vi "Script Dyn-Conf.vi"(6 "error in (no error)":errorcluster, 7 "TDX":bool[](array[boolean]), 8 "DelayuS":i32=7, 9 "VISA resource name IN":refnum<visa-resource-name>) -> (0 "error out":errorcluster, 1 "Tamaño Script":i32, 2 "Orden Transd":u64, 3 "VISA resource name OUT":refnum<visa-resource-name>)   [LabVIEW 2014, in "CAP-USB.lvlib"]
doc: "Este VI arma un array de N elementos en donde cada elemento es una linea de configuracion que luego envia al CAP-USB pasa su configuracion."
uses:
  CAP-USB.lvlib
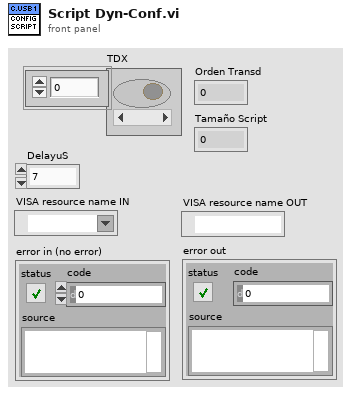
[diagram p1: front panel]
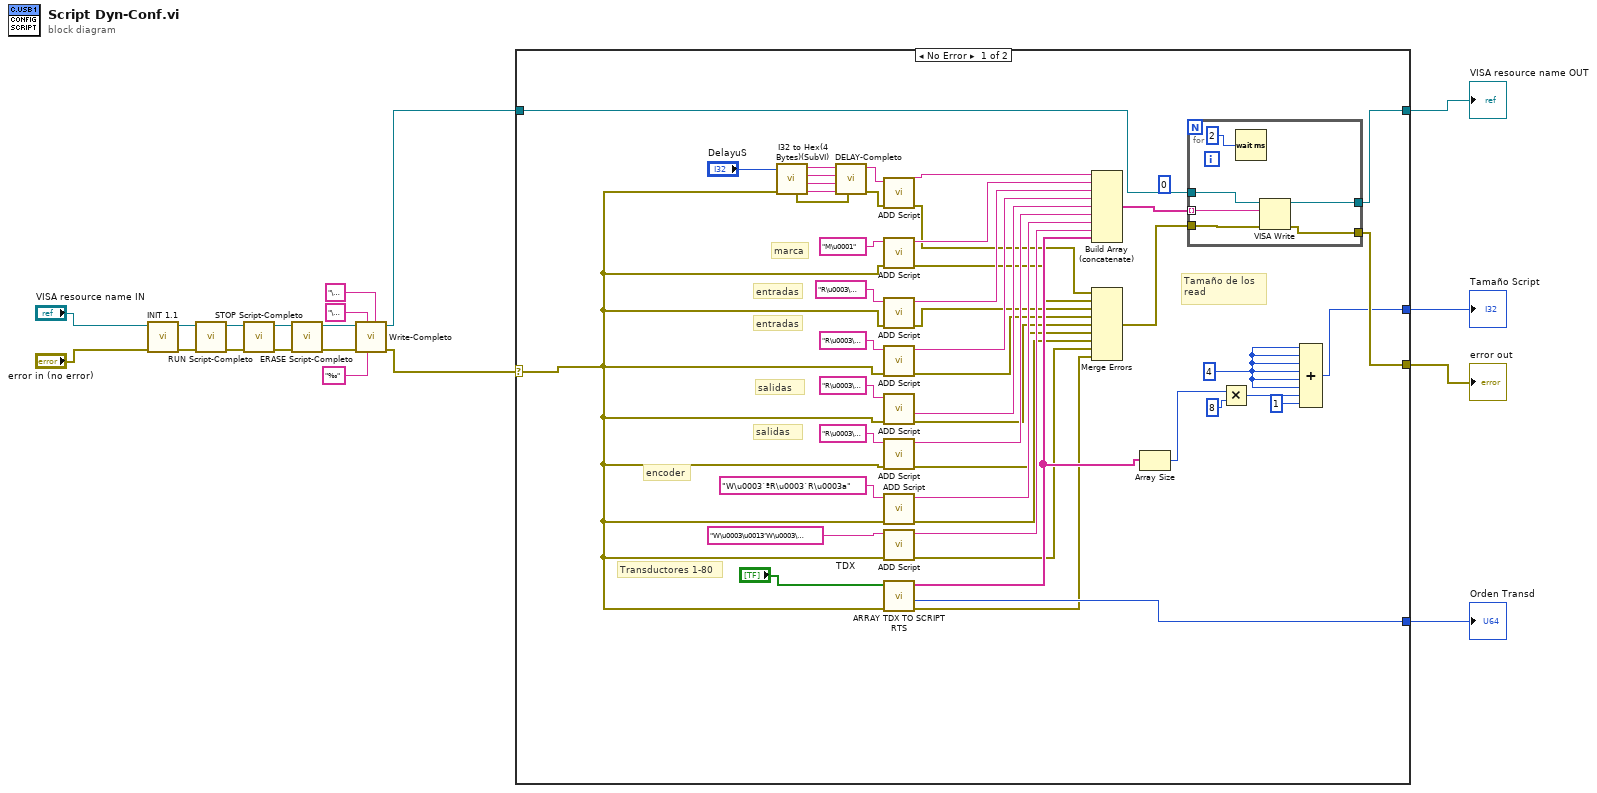
[diagram p0: block diagram]
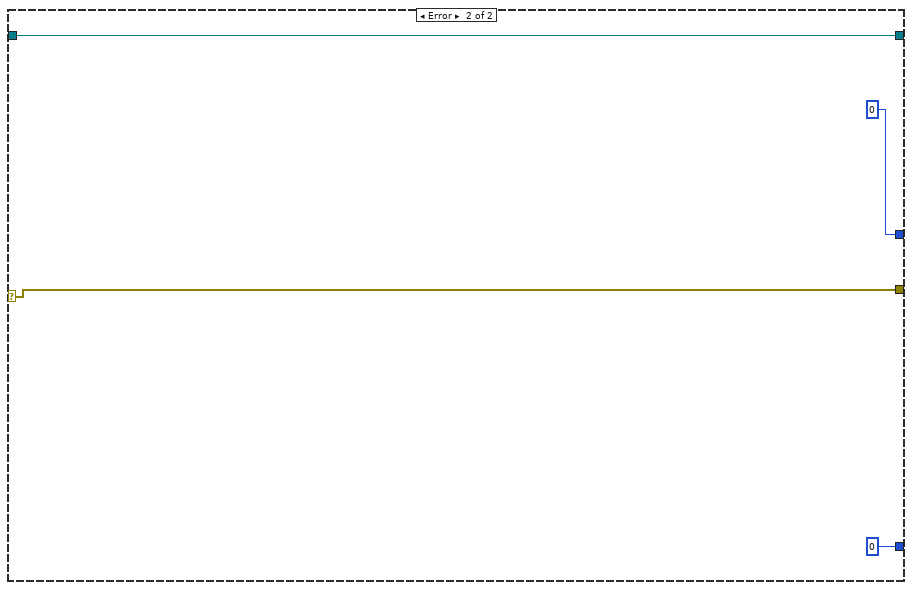
[diagram p2: hidden frame]
diagram:
  n1 = call "INIT 1.1.vi"("error in (no error)"="error in (no error)", "VISA resource name"="VISA resource name IN") -> ("error out"=w3:errorcluster, "VISA resource name out"=w4:refnum<visa-resource-name>)  [unwired: 8 in]
  n2 = call "RUN Script-Completo.vi"("error in (no error)"=w3, "VISA resource name"=w4) -> ("error out"=w10:errorcluster, "VISA resource name out"=w9:refnum<visa-resource-name>)  [unwired: 8 in]
  n3 = call "STOP Script-Completo.vi"("error in (no error)"=w10, "VISA resource name"=w9) -> ("error out"=w8:errorcluster, "VISA resource name out"=w7:refnum<visa-resource-name>)  [unwired: 8 in]
  n4 = call "ERASE Script-Completo.vi"("error in (no error)"=w8, "VISA resource name"=w7) -> ("error out"=w5:errorcluster, "VISA resource name out"=w6:refnum<visa-resource-name>)  [unwired: 8 in]
  n5 = call "Write-Completo.vi"("Low Byte"="\u0017", "Dato 8 bits"="‰", "Hi Byte"="\u0003", "error in (no error)"=w5, "VISA resource name"=w6) -> ("error out"=w1:errorcluster, "VISA resource name out"=w2:refnum<visa-resource-name>)  [unwired: 5 in]
  n6 = case shown="No Error" w1 {
    selector: w1 -> [w30 w75]
    tunnel: w2 -> [w56 w76]
    tunnel: [w55 w76] -> w19
    tunnel: [w54 w75] -> w18
    tunnel: [w52 u16 0 ("TRANSD")] -> w17
    tunnel: [w38 0] -> w16
    frame No Error {
      w40 = 4
      (unwired) 0
      # "Tamaño de los \nread"
      # "salidas"
      # "salidas"
      # "entradas"
      # "Transductores 1-80"
      # "encoder"
      # "entradas"
      # "marca"
      n7 = call "I32 to Hex(4 Bytes)(SubVI).vi"("error in (no error)"=w30, "I32"="DelayuS") -> ("BYTE 3"=w57:string, "BYTE 2"=w58:string, "BYTE1"=w59:string, "BYTE 0"=w60:string, "error out"=w32:errorcluster)  [unwired: 5 in]
      n8 = call "DELAY-Completo.vi"("error in (no error)"=w32, "Byte4(0)"=w57, "Byte3(0)"=w58, "Byte2 (0)"=w59, "Byte1 (0)"=w60) -> ("error out"=w31:errorcluster, "DelayOut"=w42:string)  [unwired: 5 in]
      n9 = call "ADD Script.vi"("error in (no error)"=w31, "Comando"=w42) -> ("error out"=w28:errorcluster, "Comando RTS"=w51:string)  [unwired: 8 in]
      n10 = call "ADD Script.vi"("error in (no error)"=w30, "Comando"="M\u0001" ("Datos a agregar")) -> ("error out"=w27:errorcluster, "Comando RTS"=w50:string)  [unwired: 8 in]
      n11 = call "ADD Script.vi"("error in (no error)"=w30, "Comando"="R\u0003\u0000" ("Datos a agregar")) -> ("error out"=w26:errorcluster, "Comando RTS"=w65:string)  [unwired: 8 in]
      n12 = call "ADD Script.vi"("error in (no error)"=w30, "Comando"="R\u0003\u0004" ("Datos a agregar")) -> ("error out"=w25:errorcluster, "Comando RTS"=w64:string)  [unwired: 8 in]
      n13 = call "ADD Script.vi"("error in (no error)"=w30, "Comando"="R\u0003\u0001" ("Datos a agregar")) -> ("error out"=w24:errorcluster, "Comando RTS"=w63:string)  [unwired: 8 in]
      n14 = call "ADD Script.vi"("error in (no error)"=w30, "Comando"="R\u0003\u0005" ("Datos a agregar")) -> ("error out"=w23:errorcluster, "Comando RTS"=w62:string)  [unwired: 8 in]
      n15 = call "ADD Script.vi"("error in (no error)"=w30, "Comando"="W\u0003`ªR\u0003`R\u0003a" ("Datos a agregar")) -> ("error out"=w22:errorcluster, "Comando RTS"=w61:string)  [unwired: 8 in]
      n16 = call "ADD Script.vi"("error in (no error)"=w30, "Comando"="W\u0003\u0013’W\u0003\u0012ð" ("Datos a agregar")) -> ("error out"=w21:errorcluster, "Comando RTS"=w34:string)  [unwired: 8 in]
      n17 = call "ARRAY TDX TO SCRIPT RTS .vi"("error in (no error)"=w30, "TDX"="TDX") -> ("error out"=w20:errorcluster, "TRANSD"=w52:u64, "SCRIPT OUT"=w36:string[])  [unwired: 7 in]
      n18 = Build Array (concatenate)(w51, w50, w65, w64, w63, w62, w61, w34, w36) -> (w49:string[])
      n19 = Merge Errors(w28, w27, w26, w25, w24, w23, w22, w21, w20) -> (w29:errorcluster)
      n20 = Array Size(array=w36) -> (size(s)=w41:i32)
      n21 = for {
        tunnel: w49 -> [w67] mode=indexing
        tunnel: w56 -> [w72]
        tunnel: w29 -> [w71]
        tunnel: [w70] -> w55
        tunnel: [w69] -> w54
        n22 = Wait (ms)(milliseconds to wait=u32 2) -> ()  [unwired: 1 out]
        n23 = VISA Write(VISA resource name=w72, write buffer=w67, error in (no error)=w71) -> (VISA resource name out=w70:refnum<visa-resource-name>, error out=w69:errorcluster)  [unwired: 1 out]
      }
      n24 = Multiply(x=w41, y=8) -> (x*y=w39:i32)
      n25 = Compound Arithmetic op=ADD(w40, w40, w40, w40, w40, w40, w39, 1 ("value")) -> (w38:i32)
    }
    frame Error {
    }
  }
  "VISA resource name OUT" <- w19
  "error out" <- w18
  "Orden Transd" <- w17
  "Tamaño Script" <- w16
